vi "addImage.vi"(8 "error in (no error)":errorcluster, 9 "number of images":i32=3, 10 "ImageData":T1, 11 "AbsorptionAnalyser in":refnum<class "AbsorptionAnalyser.lvclass">) -> (0 "error out":errorcluster, 3 "AbsorptionAnalyser out":refnum<class "AbsorptionAnalyser.lvclass">)   [LabVIEW 2009, in "Tools.lvlib" / "Imaging.lvlib" / "AbsorptionAnalyser.lvclass"]
uses:
  AbsorptionAnalyser.lvclass
  AbsorptionAnalyser.lvclass/AbsorptionAnalyser.ctl
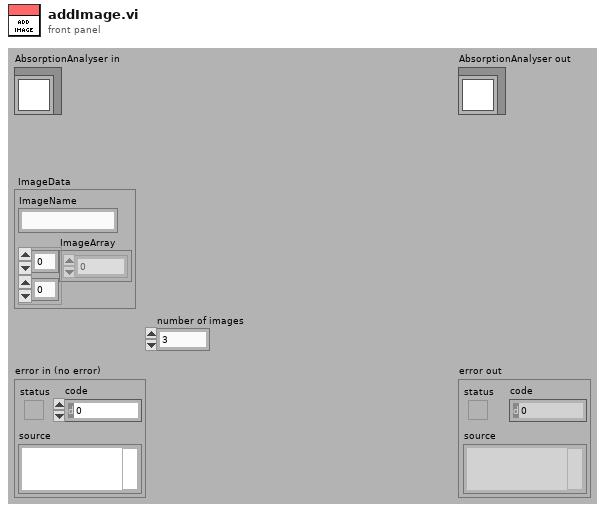
[diagram p1: front panel]
types:
  T1 = cluster{"ImageName":string, "ImageArray":sgl[][]}
  T2 = cluster{"ImageName":string, "ImageArray":sgl[][]}[]
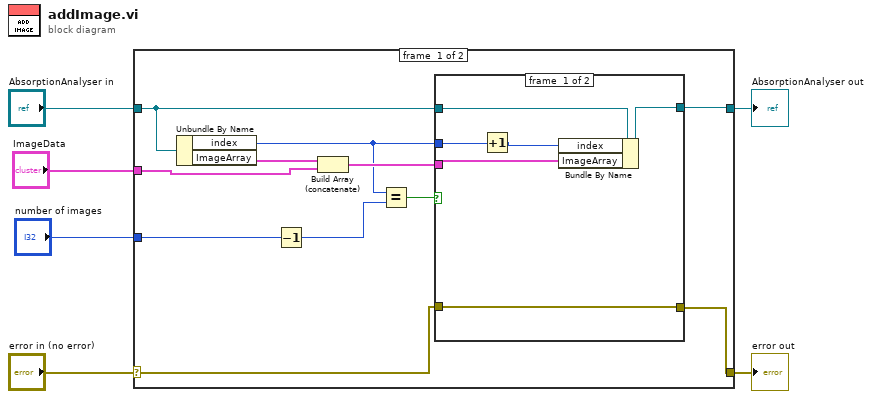
[diagram p0: block diagram]
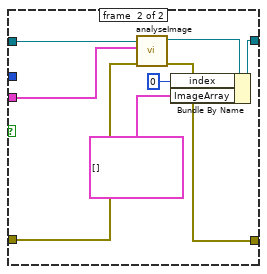
[diagram p2: hidden frame]
diagram:
  n1 = case shown="No Error" "error in (no error)" {
    selector: "error in (no error)" -> [w11 w33]
    tunnel: [w10 w33] -> w5
    tunnel: [w12 w32] -> w3
    tunnel: "AbsorptionAnalyser in" -> [w15 w32]
    tunnel: "ImageData" -> [w9 _]
    tunnel: "number of images" -> [w7 _]
    frame #0 {
      n2 = Unbundle By Name(w15) -> ("index"=w13:i32, "ImageArray"=w17:T2)
      n3 = Decrement(x=w7) -> (x-1=w8:i32)
      n4 = Build Array (concatenate)(w17, w9) -> (w14:T2)
      n5 = Equal?(x=w13, y=w8) -> (x = y?=w16:bool)
      n6 = case shown="True" w16 {
        tunnel: w15 -> [w22 w31]
        tunnel: w14 -> [w19 w28]
        tunnel: w13 -> [w23 _]
        tunnel: [w21 w26] -> w12
        tunnel: w11 -> [w18 w30]
        tunnel: [w18 w29] -> w10
        frame #0 {
          n7 = Increment(x=w23) -> (x+1=w20:i32)
          n8 = Bundle By Name(cluster=w22, "index"=w20, "ImageArray"=w19) -> (w21:refnum<class "AbsorptionAnalyser.lvclass">)
        }
        frame #1 {
          n9 = call-dynamic "analyseImage.vi"("error in (no error)"=w30, "Array"=w28, "AbsorptionAnalyser in"=w31) -> ("error out"=w29:errorcluster, "AbsorptionAnalyser out"=w27:refnum<class "AbsorptionAnalyser.lvclass">)  [unwired: 7 in]
          n10 = Bundle By Name(cluster=w27, "index"=0, "ImageArray"=T2 []) -> (w26:refnum<class "AbsorptionAnalyser.lvclass">)
        }
      }
    }
    frame #1 {
    }
  }
  "error out" <- w5
  "AbsorptionAnalyser out" <- w3
